vi "AutoGlobal.vi"() -> ()   [LabVIEW 2020]
uses:
  Arm/ArmGamePiecePreset.ctl
  Arm/ArmPositionPreset.ctl
panel:
  in  "QuickAutoDistance":dbl
  in  "QuickAutoPosition":T1=enum."Middle"
  in  "QuickAutoGamePiece":T2
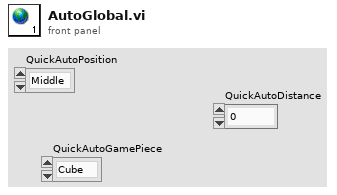
[diagram p1: front panel]
types:
  T1 = typedef "ArmPositionPreset.ctl" = enum16{"Upper", "Lower", "Middle", "Home", "Shelf", "Floor"}
  T2 = typedef "ArmGamePiecePreset.ctl" = enum16{"Cube", "Cone"}
diagram:
